vi "PH_Sixpack.constructor.vi"(0 "name":string, 2 "data in":string, 5 "error in":errorcluster) -> (14 "i ref out":refnum<vi>, 16 "data out":string, 19 "error out":errorcluster)   [LabVIEW 2014, in "PH_Sixpack.lvlib"]
doc: "six-pack controller for Trinamics stepper motor controller\n\nauthor: Max Kugler and Stefan Götte, GSI\n\nLicense Agreement for this software:\n\nCopyright (C)\nGesellschaft für Schwerionenforschung, GSI\nPlanckstr. 1\n64291 Darmstadt\nGermany\n\nContact: D.Beck@gsi.de \n\nThis program is free software; you can redistribute it and/or modify it under the terms of the \nGNU General Public License as published by the Free Software Foundation; either version 2 of \nthe license, or (at your option) any later version.\n\nThis program is distributed in the hope that it will be useful, but WITHOUT ANY WARRANTY; \nwithout even the implied warranty of MERCHANTABILITY or FITNESS FOR A PARTICULAR PURPOSE. See the GNU General License for more details (http://www.gnu.org).\n\nGesellschaft für Schwerionenforschung, GSI\nPlanckstr. 1, 64291 Darmstadt, Germany\nFor all questions and ideas contact: M.Richter@gsi.de, H.Brand@gsi.de or D.Beck@gsi.de.\nLast update: 16-JUN-2004"
uses:
  PH_Sixpack.lvlib
  PH_Sixpack.Status.ctl
  PH_Basics/PH_Stepmotor_BaseClass/PH_Stepmotor_BaseClass.lvlib
  CS_Core/CSSystem/CSSystemLib/CSSystemLib.lvlib
  PH_Basics/PH_Class/PH_Class.lvlib
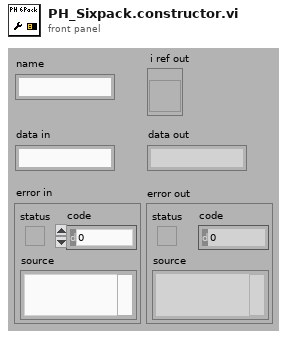
[diagram p1: front panel]
types:
  T1 = typedef "PH_Sixpack.lvlib/PH_Sixpack.Status.ctl" = enum32{"None", "Init", "Configure", "configured", "Close", "closed"}
  T2 = enum16{"SetAttribute", "GetAttribute", "CreateAttribute", "DestroyAttribute", "DestroyAllAtributes"}
  T3 = typedef "PH_Sixpack.lvlib/PH_Sixpack.i attribute.ctl" = cluster{"Information":cluster{"SixPack ID(0)":u16, "BaudRate(19200)":u16, "COM Port":enum32{"COM1", "COM2", "COM3", "COM4", "COM5", "COM6", "COM7", "COM8", "COM9"}, "HANDLE":i32}, "Serial Number":dbl, "Firmwareversion":dbl, "Axes":T4[], "Status":T1, "Axis to do a RefSearch":i32, "GUI Refs":cluster{"Information":refnum<vi>, "Serial Number":refnum<vi>, "Firmwareversion":refnum<vi>, "Status":refnum<vi>, "Axis to do a RefSearch":refnum<vi>, "Axes Configuration (Sixpack)":refnum<vi>, "Inputs":refnum<vi>, "PeriodicInterval [ms]":refnum<vi>}, "Constructor finished":bool, "Ignore Error":bool}
  T4 = typedef "PH_Sixpack.lvlib/PH_Sixpack.Axis Cluster.ctl" = cluster{"Config":T5, "To set?":cluster{"VmaxAmax":bool, "I max":bool, "VStartVminDivi":bool, "Ref Search Parameter":bool, "Stopswitch Limits":bool, "Axis Parameter":bool, "I Control":bool}}
  T5 = typedef "PH_Sixpack.lvlib/PH_Sixpack.Axis Configuration.ctl" = cluster{"VmaxAmax":T6, "I max (50%)":T7, "VStartVminDivi":T8, "Ref Search Parameter":T9, "Stopswitch Limits":T10, "Axis Parameter":T11, "I Control":T14}
  T6 = typedef "Sixpack - Driver.lvlib/VmaxAmax.ctl" = cluster{"VMax(511)":u16, "AMax(128)":u16}
  T7 = typedef "Sixpack - Driver.lvlib/PeakCurrent.ctl" = dbl
  T8 = typedef "Sixpack - Driver.lvlib/VStartVmin.ctl" = cluster{"VStart(5)":u16, "Vmin(4)":u16, "Div i (2)":enum8{"0", "1", "2", "3"}}
  T9 = typedef "Sixpack - Driver.lvlib/Ref Search Parameter.ctl" = cluster{"VRefMax(100)":u16, "DebouncingTime (22ms)":u8}
  T10 = typedef "Sixpack - Driver.lvlib/Stopswitch Limits.ctl" = cluster{"MinLeft(0)":u16, "MaxRight(1023)":u16}
  T11 = typedef "Sixpack - Driver.lvlib/Motor Parameter.ctl" = cluster{"Poslimit (6400)":u32, "P5 Bits":T12, "P6 Bits":T13}
  T12 = typedef "Sixpack - Driver.lvlib/MotorParameter_P5.ctl" = cluster{"MT_PI":bool, "MT_ROTARY":bool, "MT_AUTONULLCMD":bool, "MT_TESTNULL":bool, "MT_NULLLEFT":bool, "MT_NULLCENTRE":bool, "MT_STOPNULL":bool, "MT_FILTERSWITCH":bool}
  T13 = typedef "Sixpack - Driver.lvlib/MotorParameter_P6.ctl" = cluster{"MT_OPTIMIZEWAY":bool, "MT_FASTREF":bool, "MT_MECHREF":bool, "MT_DELAYTESTNULL":bool, "MT_STOPSOFT":bool, "MT_STOPNOREF":bool, "MT_NULLPOSITIVE":bool, "MUT_STOPFULSTEPS":bool}
  T14 = typedef "Sixpack - Driver.lvlib/Current Control.ctl" = cluster{"PowerDownDelay (500)":u16, "PowerDown (0%)":T15, "Standing (50%)":T15, "Running (75%)":T15, "Accelerating (100%)":T15}
  T15 = typedef "Sixpack - Driver.lvlib/Current.ctl" = enum8{"100%", "75%", "50%", "38%", "25%", "19%", "13%", "9%", "0%"}
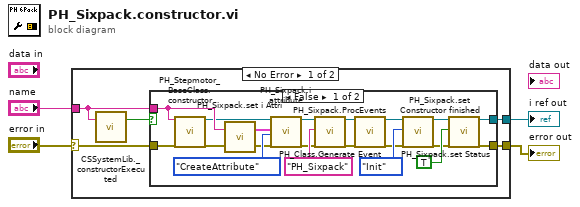
[diagram p0: block diagram]
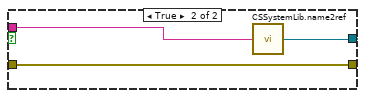
[diagram p2: hidden frame]
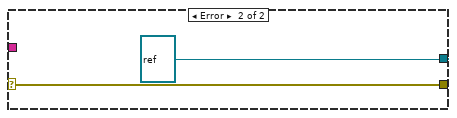
[diagram p3: hidden frame]
diagram:
  n1 = case shown="No Error" "error in" {
    selector: "error in" -> [w9 w34]
    tunnel: "name" -> [w6 _]
    tunnel: [w8 refnum<vi> refnum ("i ref out")] -> w3
    tunnel: [w7 w34] -> w2
    frame No Error {
      n2 = call "CSSystemLib._constructorExecuted.vi"("name"=w6) -> ("constructor executed?"=w5:bool)  [unwired: 18 in]
      n3 = case shown="False" w5 {
        tunnel: w9 -> [w28 w30]
        tunnel: [w27 w31] -> w8
        tunnel: [w26 w30] -> w7
        tunnel: w6 -> [w12 w32]
        frame False {
          n4 = call "PH_Stepmotor_BaseClass.constructor.vi"("name"=w12, "error in"=w28) -> ("i ref out"=w10:refnum<vi>, "error out"=w14:errorcluster)  [unwired: 15 in, 1 out]
          n5 = call "PH_Sixpack.set i Attri.vi"("error in (no error)"=w14, "Instance Name"=w12) -> ("error out"=w13:errorcluster, "i Attributes"=w11:T3)
          n6 = call "PH_Sixpack.i attribute.vi"("VI Refnum"=w10, "CLASS.i attribute"=w11, "Action"=T2."CreateAttribute", "error in (no error)"=w13) -> ("VI Refnum out"=w15:refnum<vi>, "error out"=w18:errorcluster)  [unwired: 13 in, 1 out]
          n7 = call "PH_Class.Generate Event.vi"("i ref in"=w15, "Class"="PH_Sixpack", "error in (no error)"=w18) -> ("i ref out"=w16:refnum<vi>, "error out"=w17:errorcluster)  [unwired: 15 in]
          n8 = call "PH_Sixpack.ProcEvents.vi"("i ref in"=w16, "error in"=w17) -> ("i ref out"=w20:refnum<vi>, "error out"=w19:errorcluster)  [unwired: 16 in]
          n9 = call "PH_Sixpack.set Status.vi"("VI in"=w20, "Status"=PH_Sixpack.Status."Init", "error in (no error)"=w19) -> ("VI out"=w23:refnum<vi>, "error out"=w21:errorcluster)  [unwired: 15 in]
          n10 = call "PH_Sixpack.set Constructor finished.vi"("VI in"=w23, "Constructor finished?"=TRUE, "error in (no error)"=w21) -> ("VI out"=w27:refnum<vi>, "error out"=w26:errorcluster)  [unwired: 15 in]
        }
        frame True {
          n11 = call "CSSystemLib.name2ref.vi"("name"=w32) -> ("obj refnum"=w31:refnum<vi>)
        }
      }
    }
    frame Error {
    }
  }
  "i ref out" <- w3
  "error out" <- w2
